vi "Kinect Find Blobs.vi"(0 "Image Src":T2, 1 "Range":cluster{"Lower value":sgl, "Upper value":sgl}={"Lower value"=10.0, "Upper value"=32768.0} {"Upper value" format="%.2f"; "Lower value" format="%.2f"}, 5 "Selection Values":T4(array[cluster]) {"Measurement Parameter" items=["Center of Mass X", "Center of Mass Y", "First Pixel X", "First Pixel Y", "Bounding Rect Left", "Bounding Rect Top", "Bounding Rect Right", "Bounding Rect Bottom", "Max Feret Diameter Start X", "Max Feret Diameter Start Y", "Max Feret Diameter End X", "Max Feret Diameter End Y", "Max Horiz. Segment Length Left", "Max Horiz. Segment Length Right", "Max Horiz. Segment Length Row", "-", "Bounding Rect Width", "Bounding Rect Height", "Bounding Rect Diagonal", "Perimeter", "Convex Hull Perimeter", "Holes' Perimeter", "Max Feret Diameter", "Equivalent Ellipse Major Axis", "Equivalent Ellipse Minor Axis", "Equivalent Ellipse Minor Axis (Feret)", "Equivalent Rect Long Side", "Equivalent Rect Short Side", "Equivalent Rect Diagonal", "Equivalent Rect Short Side (Feret)", "Average Horiz. Segment Length", "Average Vert. Segment Length", "Hydraulic Radius", "Waddel Disk Diameter", "-", "Area", "Holes' Area", "Particle & Holes' Area", "Convex Hull Area", "Image Area", "-", "Number of Holes", "Number of Horiz. Segments", "Number of Vert. Segments", "-", "Orientation", "Max Feret Diameter Orientation", "-", "% Area/Image Area", "% Area/(Particle & Holes' Area)", "Ratio of Equivalent Ellipse Axes", "Ratio of Equivalent Rect Sides", "-", "Elongation Factor", "Compactness Factor", "Heywood Circularity Factor", "Type Factor", "-", "Sum X", "Sum Y", "Sum XX", "Sum XY", "Sum YY", "Sum XXX", "Sum XXY", "Sum XYY", "Sum YYY", "-", "Moment of Inertia XX", "Moment of Inertia XY", "Moment of Inertia YY", "Moment of Inertia XXX", "Moment of Inertia XXY", "Moment of Inertia XYY", "Moment of Inertia YYY", "Norm. Moment of Inertia XX", "Norm. Moment of Inertia XY", "Norm. Moment of Inertia YY", "Norm. Moment of Inertia XXX", "Norm. Moment of Inertia XXY", "Norm. Moment of Inertia XYY", "Norm. Moment of Inertia YYY", "Hu Moment 1", "Hu Moment 2", "Hu Moment 3", "Hu Moment 4", "Hu Moment 5", "Hu Moment 6", "Hu Moment 7"]; "Range Lower Value" format="%.2f"; "Range Upper Value" format="%.2f"}, 7 "# Points in Spline":i32=50, 9 "degree":i32=3, 11 "Number of Erosion":i32=10, 12 "Spline Style":u16(ring)=2 items=["equally spaced", "chord length", "centripetal"]) -> (4 "Masked Image Out":T2, 6 "Particle Reports (Pixels)":T1(array[cluster]) {"Orientation" format="%.2f"; "Dimensions"."Height" format="%.2f"; "Dimensions"."Width" format="%.2f"; "Center of Mass"."Y" format="%.2f"; "Center of Mass"."X" format="%.2f"; "Bounding Rect"."Bottom" format="%.2f"; "Bounding Rect"."Right" format="%.2f"; "Bounding Rect"."Top" format="%.2f"; "Bounding Rect"."Left" format="%.2f"; "Number of Holes" format="%.2f"; "Area" format="%.2f"})   [LabVIEW 2011]
uses:
  <vilib>/vision/Image Controls.llb/IMAQ Image.ctl
  <vilib>/vision/NI_Vision_Development_Module.lvlib
  <vilib>/Analysis/NI_AALPro.lvlib
panel:
  out "Number of Particles":i32
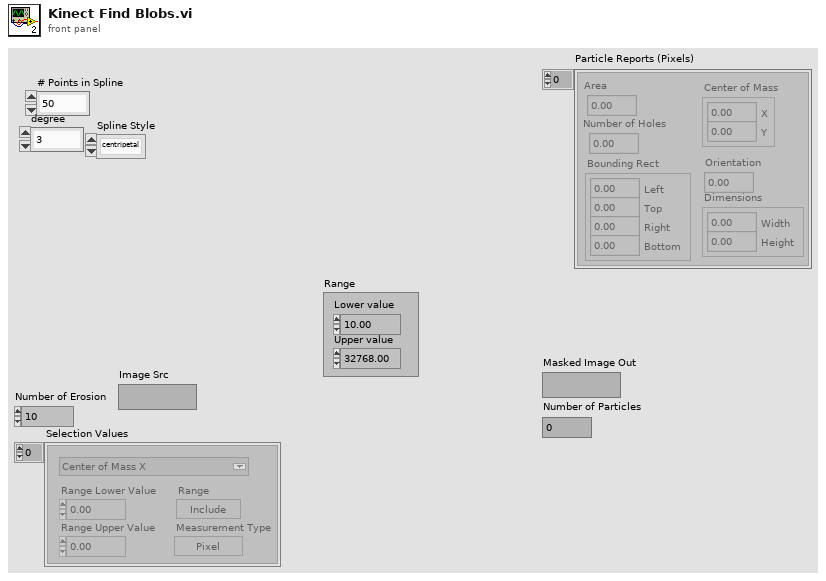
[diagram p1: front panel]
types:
  T1 = cluster{"Area":dbl, "Number of Holes":dbl, "Bounding Rect":cluster{"Left":dbl, "Top":dbl, "Right":dbl, "Bottom":dbl}, "Center of Mass":cluster{"X":dbl, "Y":dbl}, "Orientation":dbl, "Dimensions":cluster{"Width":dbl, "Height":dbl}}[]
  T2 = typedef "IMAQ Image.ctl" = refnum<image>
  T3 = typedef "Particle Parameters" = i32
  T4 = cluster{"Measurement Parameter":T3, "Range Lower Value":dbl, "Range Upper Value":dbl, "Range":bool, "Measurement Type":bool}[]
  T5 = typedef "Image Type" = u32
  T6 = typedef "ROI Descriptor" = cluster{"Global Rectangle":i32[], "Contours":cluster{"ID":enum32{"External", "Internal"}, "Type":u32, "Coordinates":i32[]}[]}
  T7 = cluster{"ID":enum32{"External", "Internal"}, "Type":u32, "Coordinates":i32[]}[]
  T8 = cluster{"ID":enum32{"External", "Internal"}, "Type":u32, "Coordinates":i32[]}
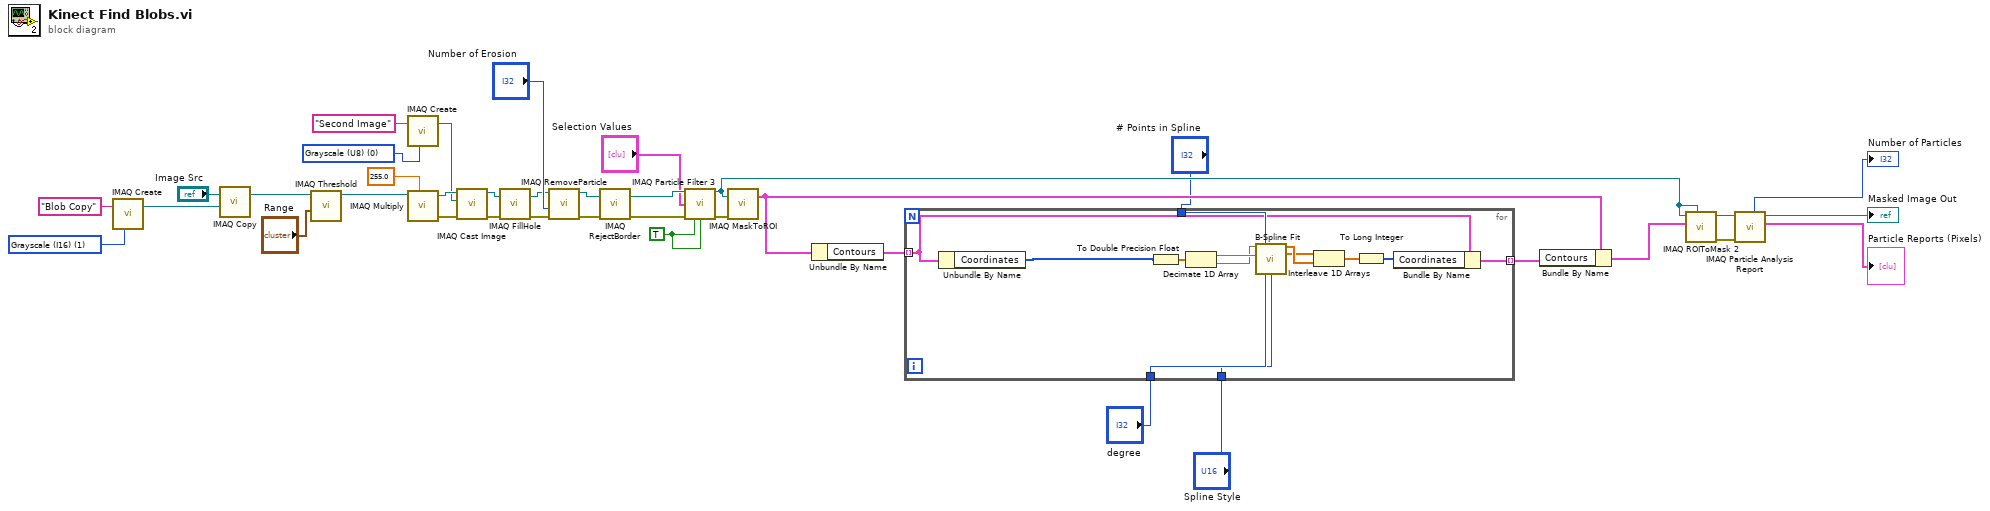
[diagram p0: block diagram]
diagram:
  w17 = T5 1 items=["Grayscale (U8)", "Grayscale (I16)", "Grayscale (SGL)", "Complex (CSG)", "RGB (U32)", "HSL (U32)", "RGB (U64)", "Grayscale (U16)"] ("Image Type")
  w25 = TRUE ("Fill Holes? (F)")
  w33 = T5 0 items=["Grayscale (U8)", "Grayscale (I16)", "Grayscale (SGL)", "Complex (CSG)", "RGB (U32)", "HSL (U32)", "RGB (U64)", "Grayscale (U16)"] ("Image Type")
  n1 = call "IMAQ Create"("Image Name"="Blob Copy", "Image Type"=w17) -> ("New Image"=w18:T2)  [unwired: 3 in, 1 out]
  n2 = call "IMAQ Copy"("Image Dst"=w18, "Image Src"="Image Src") -> ("Image Dst Out"=w19:T2)  [unwired: 4 in, 1 out]
  n3 = call "IMAQ Threshold"("Range"="Range", "Image Src"=w19) -> ("Image Dst Out"=w37:T2)  [unwired: 8 in, 1 out]
  n4 = call "IMAQ Create"("Image Name"="Second Image", "Image Type"=w33) -> ("New Image"=w32:T2)  [unwired: 3 in, 1 out]
  n5 = call "IMAQ Multiply"("Image Src A"=w37, "Constant"=sgl 255.0) -> ("Image Dst Out"=w35:T2, "error out"=w36:errorcluster)  [unwired: 5 in]
  n6 = call "IMAQ Cast Image"("error in (no error)"=w36, "Image Dst"=w32, "Image Src"=w35) -> ("error out"=w22:errorcluster, "Image Dst Out"=w23:T2)  [unwired: 7 in]
  n7 = call "IMAQ FillHole"("error in (no error)"=w22, "Image Src"=w23) -> ("error out"=w21:errorcluster, "Image Dst Out"=w24:T2)  [unwired: 4 in]
  n8 = call "IMAQ RemoveParticle"("error in (no error)"=w21, "Number of Erosion"="Number of Erosion", "Image Src"=w24) -> ("error out"=w29:errorcluster, "Image Dst Out"=w9:T2)  [unwired: 7 in]
  n9 = call "IMAQ RejectBorder"("error in (no error)"=w29, "Image Src"=w9) -> ("error out"=w26:errorcluster, "Image Dst Out"=w28:T2)  [unwired: 4 in]
  n10 = call "IMAQ Particle Filter 3"("Image Src"=w28, "Selection Values"="Selection Values", "error in (no error)"=w26, "Reject Border? (F)"=w25, "Fill Holes? (F)"=w25) -> ("Image Dst Out"=w8:T2, "error out"=w12:errorcluster)  [unwired: 4 in, 5 out]
  n11 = call "IMAQ MaskToROI"("Image"=w8, "error in (no error)"=w12) -> ("ROI Descriptor"=w7:T6)  [unwired: 5 in, 2 out]
  n12 = Unbundle By Name(w7) -> ("Contours"=w4:T7)
  n13 = for {
    tunnel: "# Points in Spline" -> [w51]
    tunnel: w4 -> [w46] mode=indexing
    tunnel: "degree" -> [w48]
    tunnel: "Spline Style" -> [w47]
    tunnel: [w44] -> w1 mode=indexing
    n14 = Unbundle By Name(w46) -> ("Coordinates"=w39:i32[])
    n15 = To Double Precision Float(number=w39) -> (double precision float=w42:dbl[])
    n16 = Decimate 1D Array(w42) -> (w41:dbl[], w40:dbl[])
    n17 = call <vilib>:"B-Spline Fit.vi"("Y"=w40, "# of control points"=w51, "X"=w41, "degree"=w48, "parameter selection"=w47) -> ("Best BSpline Fit Y"=w50:dbl[], "Best BSpline Fit X"=w49:dbl[])  [unwired: 7 in, 2 out]
    n18 = Interleave 1D Arrays(w49, w50) -> (w45:dbl[])
    n19 = To Long Integer(number=w45) -> (32bit integer=w43:i32[])
    n20 = Bundle By Name(cluster=w46, "Coordinates"=w43) -> (w44:T8)
  }
  n21 = Bundle By Name(cluster=w7, "Contours"=w1) -> (w6:T6)
  n22 = call "IMAQ ROIToMask 2"("Image Model"=w8, "ROI Descriptor"=w6, "Image"=w8) -> ("error out"=w11:errorcluster, "Image Out"=w10:T2)  [unwired: 6 in, 1 out]
  n23 = call "IMAQ Particle Analysis Report"("error in (no error)"=w11, "Image"=w10) -> ("Particle Reports (Pixels)"=→"Particle Reports (Pixels)":T1, "Image Out (duplicate)"=→"Masked Image Out":T2, "Number of Particles"=→"Number of Particles":i32)  [unwired: 4 in, 3 out]
